vi "ClassPanel.vi"(8 "error in (no error)":errorcluster caption="entrée d'erreur (pas d'erreur)", 11 "EG_G5210.lvclass":refnum<class "EG_G5210.lvclass">) -> (0 "error out":errorcluster caption="sortie d'erreur", 3 "EG_G5210.lvclass Out":refnum<class "EG_G5210.lvclass">)   [LabVIEW 2010, in "EG_G5210.lvclass"]
uses:
  EG_G5210.lvclass
  BaseDevice/BaseDevice.lvclass
panel:
  out "Sensitivity":u16(ring)=13 items=["100 nV", "300 nV", "1 µV", "3 µV", "10 µV", "30 µV", "100µV", "300 µV", "1 mV", "3 mV", "10 mV", "30 mV", "100 mV", "300 mV", "1 V", "3 V"]
  out "Phase":dbl=1000.0 caption="Phase (°)" min=0.0 step=0.1 format="%#.1f"
  out "MAG":dbl=1000.0 caption="MAG (V)" min=0.0 step=0.1 format="%#.1f"
  out "UNLCK":bool caption="SpexMov"
  out "X":dbl=1000.0 caption="X (V)" min=0.0 step=0.1 format="%#.1f"
  in  "Stop":bool
  out "Init Program":bool
  out "OVLD":bool caption="SpexMov"
  in  "Update":bool caption="stopSpectro"
  out "Y":dbl=1000.0 caption="Y (V)" min=0.0 step=0.1 format="%#.1f"
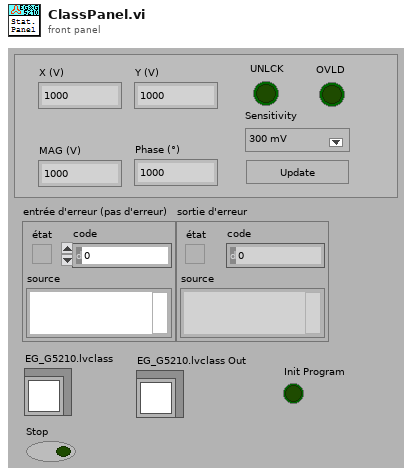
[diagram p1: front panel]
types:
  T1 = enum16{"X Output", "Y Output", "X and Y Output", "Mag", "Phase", "Mag & Phase", "X,Y,Mag & Phase", "Noise", "Aux In 1", "Aux In 2", "Aux In 3", "Aux In 4"}
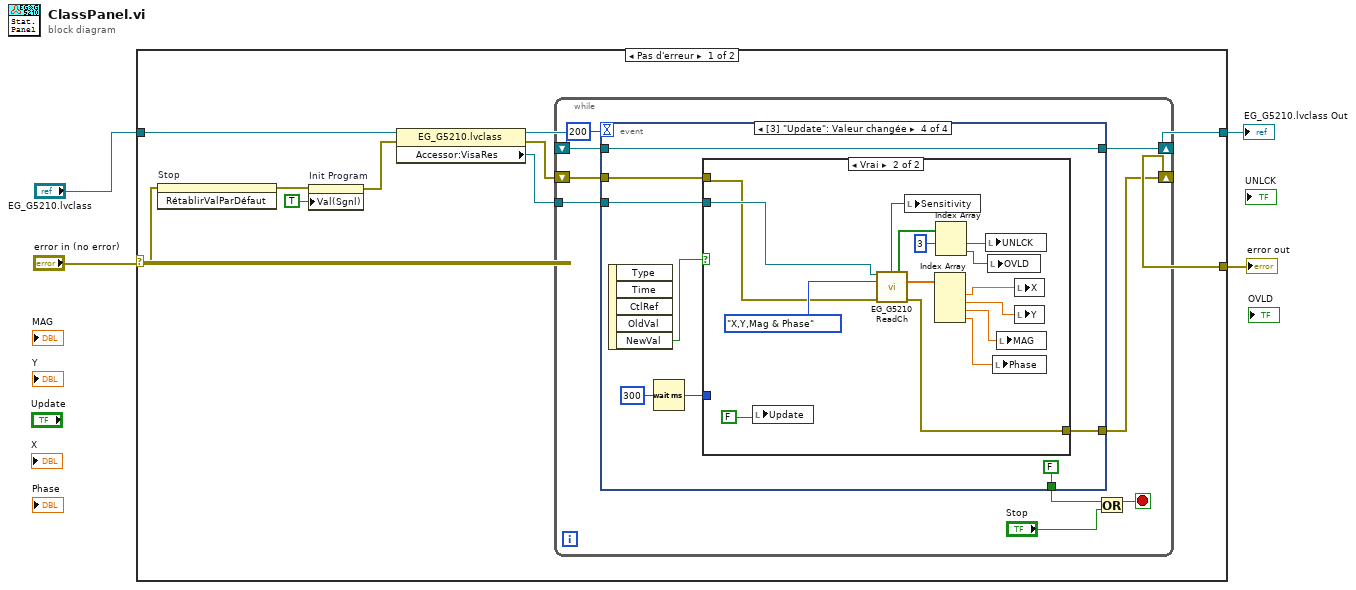
[diagram p0: block diagram]
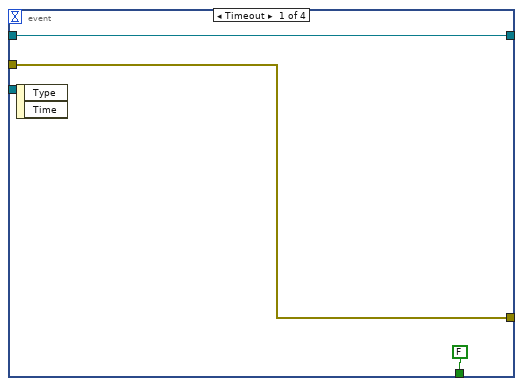
[diagram p2: hidden frame]
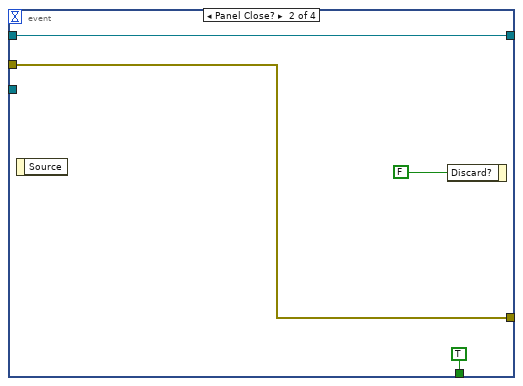
[diagram p3: hidden frame]
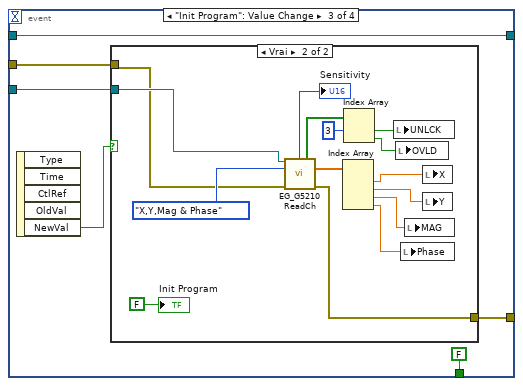
[diagram p4: hidden frame]
diagram:
  n1 = case shown="Pas d'erreur" "error in (no error)" {
    selector: "error in (no error)" -> [w9 w78]
    tunnel: [w14 w78] -> w3
    tunnel: "EG_G5210.lvclass" -> [w13 w77]
    tunnel: [w10 w77] -> w1
    frame No Error {
      n2 = invoke on="Stop" class="Bool (strict)" method="RétablirValParDéfaut"(error in=w9) -> (error out=w8:errorcluster)  [unwired: 2 in, 2 out]
      n3 = property on="Init Program" class="Bool (strict)"(error in=w8, "Val(Sgnl)"=TRUE ("Valeur (Signalisation)")) -> (error out=w7:errorcluster)  [unwired: 1 in, 1 out]
      n4 = property class="EG_G5210.lvclass"(reference=w13, error in=w7) -> (reference out=w12:refnum<class "EG_G5210.lvclass">, error out=w5:errorcluster, "Accessor:VisaRes"=w6:refnum<visa-resource-name>)
      n5 = while {
        shift-right: [w21] -> w14
        shift-left: w5 -> [w22]
        tunnel: w6 -> [w18]
        shift-right: [w17] -> w10
        shift-left: w12 -> [w20]
        stop <- w16 stop-if-true
        n6 = event shown="[3] \"Update\": Valeur changée" {
          selector: _ -> [_ _ _ _]
          dyn-events: _ -> [_ _ _ _]
          timeout: 200 -> [_ _ _ _]
          tunnel: w22 -> [w24 w28 w34 w59]
          tunnel: [w24 w28 w33 w58] -> w21
          tunnel: w20 -> [w25 w27 w32 w57]
          tunnel: [FALSE TRUE FALSE FALSE] -> w19
          tunnel: [w25 w27 w32 w57] -> w17
          tunnel: w18 -> [_ _ w35 w60]
          event Timeout {
            n7 = event-data() -> ()  [unwired: 1 in, 2 out]
          }
          event Panel Close? {
            n8 = event-data() -> ()  [unwired: 1 in, 1 out]
            n9 = event-data("Discard?"=FALSE ("Rejeter ?")) -> ()  [unwired: 1 in, 1 out]
          }
          event "Init Program": Value Change {
            n10 = event-data() -> ("NewVal"=w36:bool)  [unwired: 1 in, 4 out]
            n11 = case shown="Vrai" w36 {
              tunnel: w35 -> [_ w51]
              tunnel: w34 -> [w37 w46]
              tunnel: [w37 w48] -> w33
              frame False {
              }
              frame True {
                n12 = call <userlib>:"EG_G5210 ReadCh.vi"("VISA Rsrc"=w51, "Channel"=T1."X,Y,Mag & Phase", "error in (no error)"=w46) -> ("Sensitivity"=→"Sensitivity":u16, "Status Byte"=w45:bool[], "Outputs"=w47:dbl[], "error out"=w48:errorcluster)  [unwired: 5 in, 4 out]
                n13 = Index Array(array=w47) -> (element #1=w41:dbl, element #2=w40:dbl, element #3=w39:dbl, element #4=w38:dbl)  [unwired: 4 in]
                n14 = Index Array(array=w45, index #1=3 ("indice")) -> (element #1=w43:bool, element #2=w42:bool)  [unwired: 1 in]
                n15 = local write "UNLCK"(w43) -> ()
                n16 = local write "OVLD"(w42) -> ()
                n17 = local write "Phase"(w38) -> ()
                n18 = local write "MAG"(w39) -> ()
                n19 = local write "X"(w41) -> ()
                n20 = local write "Y"(w40) -> ()
                "Init Program" <- FALSE
              }
            }
          }
          event "Update": Value Change {
            n21 = event-data() -> ("NewVal"=w55:bool)  [unwired: 1 in, 4 out]
            n22 = Wait (ms)(milliseconds to wait=u32 300 ("attente (ms)")) -> (millisecond timer value=w54:u32)
            n23 = case shown="Vrai" w55 {
              tunnel: w60 -> [_ w76]
              tunnel: w59 -> [w61 w72]
              tunnel: [w61 w74] -> w58
              tunnel: w54 -> [_ _]
              frame False {
              }
              frame True {
                n24 = local write "Update"(FALSE) -> ()
                n25 = call <userlib>:"EG_G5210 ReadCh.vi"("VISA Rsrc"=w76, "Channel"=T1."X,Y,Mag & Phase", "error in (no error)"=w72) -> ("Sensitivity"=w63:u16, "Status Byte"=w71:bool[], "Outputs"=w73:dbl[], "error out"=w74:errorcluster)  [unwired: 5 in, 4 out]
                n26 = local write "Sensitivity"(w63) -> ()
                n27 = Index Array(array=w73) -> (element #1=w67:dbl, element #2=w66:dbl, element #3=w65:dbl, element #4=w64:dbl)  [unwired: 4 in]
                n28 = Index Array(array=w71, index #1=3 ("indice")) -> (element #1=w69:bool, element #2=w68:bool)  [unwired: 1 in]
                n29 = local write "UNLCK"(w69) -> ()
                n30 = local write "OVLD"(w68) -> ()
                n31 = local write "Phase"(w64) -> ()
                n32 = local write "MAG"(w65) -> ()
                n33 = local write "X"(w67) -> ()
                n34 = local write "Y"(w66) -> ()
              }
            }
          }
        }
        n35 = Or(x=w19, y="Stop") -> (x .or. y?=w16:bool)
      }
    }
    frame Error {
    }
  }
  "error out" <- w3
  "EG_G5210.lvclass Out" <- w1
